vi "Create Enqueuer References.vi"(8 "error in (no error)":errorcluster, 11 "Owner":refnum<vi>) -> (0 "error out":errorcluster, 2 "Request-Enqueuers":T2, 3 "API-Requests":T1)   [LabVIEW 2018, in "Scripting.lvlib" / "Actor.lvlib" / "Actor.lvclass"]
uses:
  Actor.lvclass
  Request-Enqueuers.ctl
  Get State.ctl
  State.ctl
  Stop.ctl
  API-Requests.ctl
  Launched.ctl
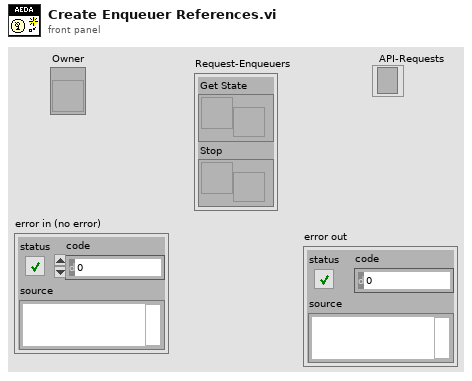
[diagram p1: front panel]
types:
  T1 = typedef "Scripting.lvlib/Actor.lvlib/Actor.lvclass/API-Requests.ctl" = refnum<event-registration>
  T2 = typedef "Scripting.lvlib/Actor.lvlib/Actor.lvclass/Request-Enqueuers.ctl" = cluster{"Get State":refnum<user-event>, "Stop":refnum<user-event>}
  T3 = typedef "Scripting.lvlib/Actor.lvlib/Actor.lvclass/Launched.ctl" = cluster{"Owner":refnum<vi>}
  T4 = typedef "Scripting.lvlib/Actor.lvlib/Actor.lvclass/Get State.ctl" = cluster{"Reply":refnum<user-event>}
  T5 = typedef "Scripting.lvlib/Actor.lvlib/Actor.lvclass/Stop.ctl" = cluster{"Type":enum16{"Normal", "Emergency"}}
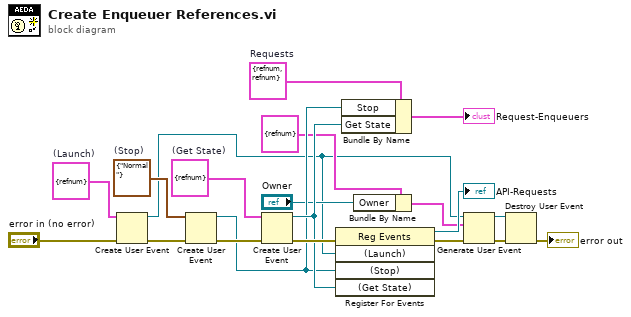
[diagram p0: block diagram]
diagram:
  w15 = T3 {"Owner"=refnum}  # (Launch)
  w17 = T4 {"Reply"=refnum}  # (Get State)
  w19 = T5 {"Type"=enum."Normal"}  # (Stop)
  w20 = T2 {"Get State"=refnum, "Stop"=refnum}  # Requests
  n1 = Create User Event(user event datatype=w15, error in="error in (no error)") -> (user event=w4:refnum<user-event>, error out=w3:errorcluster)
  n2 = Create User Event(user event datatype=w19, error in=w3) -> (user event=w10:refnum<user-event>, error out=w12:errorcluster)
  n3 = Create User Event(user event datatype=w17, error in=w12) -> (user event=w14:refnum<user-event>, error out=w16:errorcluster)
  n4 = register-events(error in=w16, w4, w10, w14) -> (reference out=→"API-Requests":refnum<event-registration>, error out=w1:errorcluster)  [unwired: 1 in]
  n5 = Bundle By Name(cluster=w20, "Stop"=w10, "Get State"=w14) -> (→"Request-Enqueuers":T2)
  n6 = Bundle By Name(cluster=T3 {"Owner"=refnum} ("event data"), "Owner"="Owner") -> (w5:T3)
  n7 = Generate User Event(user event=w4, event data cluster=w5, error in=w1) -> (user event out=w7:refnum<user-event>, error out=w6:errorcluster)  [unwired: 1 in]
  n8 = Destroy User Event(user event=w7, error in=w6) -> (error out=→"error out":errorcluster)
